vi "Open Config Path.vi"() -> (0 "error out":errorcluster, 3 "cfg_ref out":T1)   [LabVIEW 2013]
uses:
  <vilib>/Utility/config.llb/Config Data RefNum.ctl
  <vilib>/Utility/config.llb/NI_LVConfig.lvlib
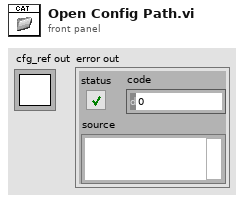
[diagram p1: front panel]
types:
  T1 = typedef "NI_LVConfig.lvlib/Config Data RefNum.ctl" = refnum<k1>
  T2 = enum16{"open", "replace", "create", "open or create", "replace or create", "replace or create with confirmation"}
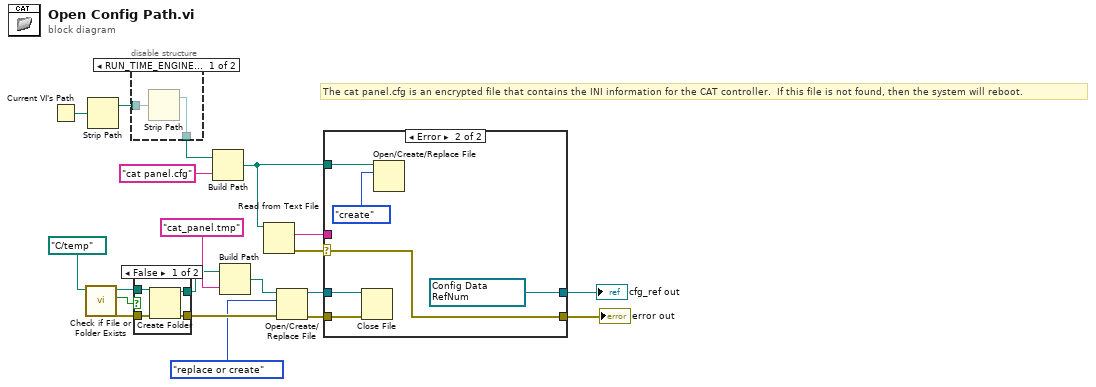
[diagram p0: block diagram]
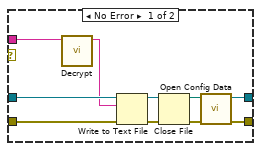
[diagram p2: hidden frame]
diagram:
  # "The cat panel.cfg is an encrypted file that contains the INI information for the CAT controller.  If this file is not found, then the system will reboot."
  n1 = Current VI's Path() -> (path=w19:path)
  n2 = call <vilib>:"Check if File or Folder Exists.vi"("path"=path "C:/temp") -> ("error out"=w12:errorcluster, "file or folder exists?"=w10:bool, "dup path"=w11:path)  [unwired: 8 in]
  n3 = Strip Path(path=w19) -> (stripped path=w18:path)  [unwired: 1 out]
  n4 = disable-structure shown="RUN_TIME_ENGINE==True" {
    disable-tunnel: w18 -> [w22 w23]
    disable-tunnel: [w21 w23] -> w17
    frame condition #0 {
      n5 = Strip Path(path=w22) -> (stripped path=w21:path)  [unwired: 1 out]
    }
    frame condition #1 (active) {
    }
  }
  n6 = case shown="False" w10 {
    tunnel: w11 -> [w27 w29]
    tunnel: w12 -> [w26 w28]
    tunnel: [w25 w29] -> w15
    tunnel: [w24 w28] -> w13
    frame False {
      n7 = Create Folder(path (use dialog)=w27, error in=w26) -> (created path=w25:path, error out=w24:errorcluster)  [unwired: 1 in, 1 out]
    }
    frame True {
    }
  }
  n8 = Build Path(base path=w17, name or relative path="cat panel.cfg") -> (appended path=w3:path)
  n9 = Build Path(base path=w15, name or relative path="cat_panel.tmp") -> (appended path=w14:path)
  n10 = Read from Text File(file (use dialog)=w3) -> (text=w4:string, error out=w5:errorcluster)  [unwired: 3 in, 2 out]
  n11 = Open/Create/Replace File(file path (use dialog)=w14, error in=w13, operation (0:open)=T2."replace or create") -> (refnum out=w7:refnum<file>, error out=w6:errorcluster)  [unwired: 3 in, 1 out]
  n12 = case shown="Error" w5 {
    selector: w5 -> [_ w41]
    tunnel: w3 -> [_ w44]
    tunnel: w4 -> [w33 _]
    tunnel: w7 -> [w39 w43]
    tunnel: w6 -> [w34 w42]
    tunnel: [w31 w41] -> w2
    tunnel: [w30 w40] -> w1
    frame No Error {
      n13 = call "Decrypt.vi"("String"=w33) -> ("Output String"=w32:string)  [unwired: 10 in]
      n14 = Write to Text File(file (use dialog)=w39, text=w32, error in=w34) -> (refnum out=w38:refnum<file>, error out=w37:errorcluster)  [unwired: 1 in, 1 out]
      n15 = Close File(refnum=w38, error in=w37) -> (path=w36:path, error out=w35:errorcluster)
      n16 = call <vilib>:"Open Config Data.vi"("error in (no error)"=w35, "configuration file path"=w36) -> ("error out"=w31:errorcluster, "refnum"=w30:T1)  [unwired: 7 in, 1 out]
    }
    frame Error {
      w40 = T1 refnum items=["config data"] ("refnum")
      n17 = Close File(refnum=w43, error in=w42) -> ()  [unwired: 2 out]
      n18 = Open/Create/Replace File(file path (use dialog)=w44, operation (0:open)=T2."create") -> ()  [unwired: 4 in, 3 out]
    }
  }
  "error out" <- w2
  "cfg_ref out" <- w1
